vi "Queue Out Unitest.vi"(8 "error in":errorcluster, 11 "?":T1) -> (0 "error out":errorcluster, 3 "Quee Out":refnum<queue>)   [LabVIEW 2025]
uses:
  REF Enum Unitest.ctl
  support/Message Queue/LAB-IQ Message Queue.lvlib
  support/Message Queue/Message Cluster.ctl
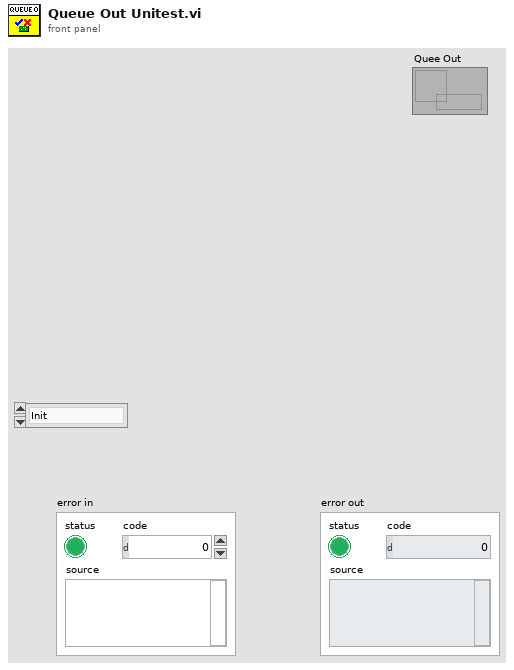
[diagram p1: front panel]
types:
  T1 = typedef "REF Enum Unitest.ctl" = enum16{"Init", "UI Loop", "LOAD COM LOOP", "HEAVE MOTOR COM LOOP", "SWAY MOTOR COM LOOP", "RAMP MOTOR COM LOOP", "TEMPERATURE COM LOOP", "HUMIDITY COM PORT", "ECR PORT", "MONITOR LOOP", "PROGRAM LOOP", "LOAD PID", "REPORT", "ACOUSTIC"}
  T2 = typedef "LAB-IQ Message Queue.lvlib/All Message Queues.ctl" = cluster{"UI Loop":refnum<queue>, "LOAD COM LOOP":refnum<queue>, "HEAVE MOTOR COM LOOP":refnum<queue>, "SWAY MOTOR COM LOOP":refnum<queue>, "RAMP MOTOR COM LOOP":refnum<queue>, "TEMPERATURE COM LOOP":refnum<queue>, "HUMIDITY COM PORT":refnum<queue>, "ECR PORT":refnum<queue>, "MONITOR LOOP":refnum<queue>, "PROGRAM LOOP":refnum<queue>, "LOAD PID":refnum<queue>, "REPORT":refnum<queue>, "ACOUSTIC":refnum<queue>}
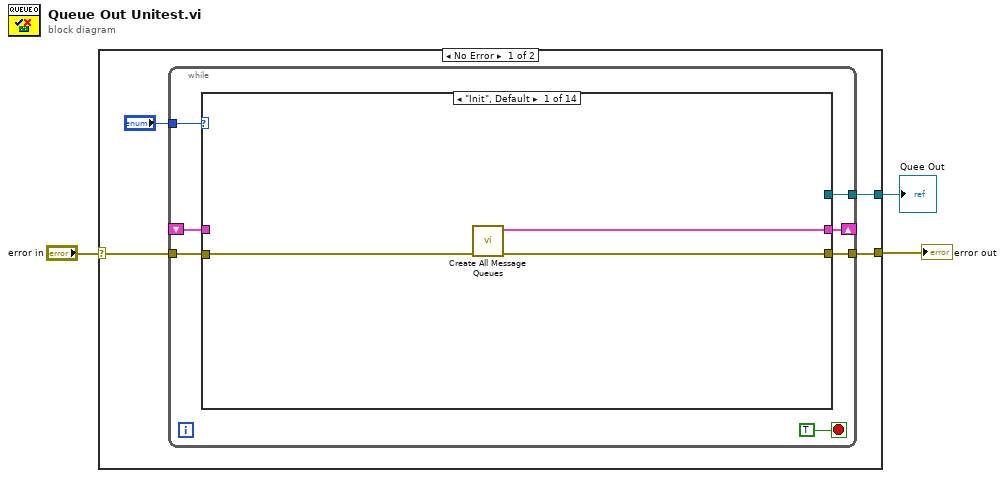
[diagram p0: block diagram]
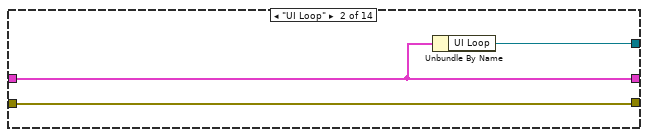
[diagram p2: hidden frame]
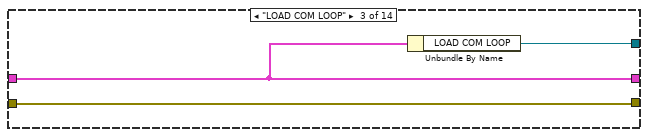
[diagram p3: hidden frame]
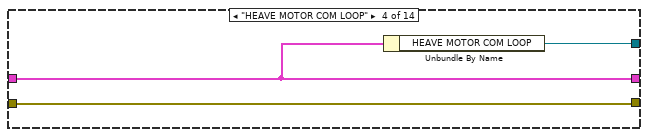
[diagram p4: hidden frame]
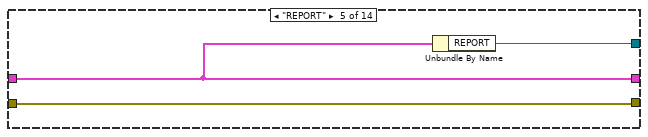
[diagram p5: hidden frame]
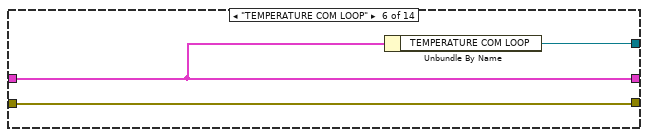
[diagram p6: hidden frame]
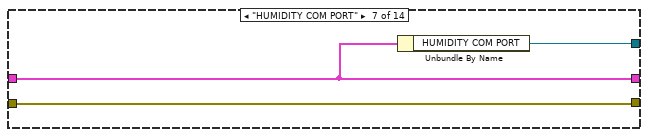
[diagram p7: hidden frame]
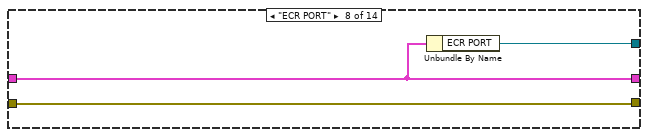
[diagram p8: hidden frame]
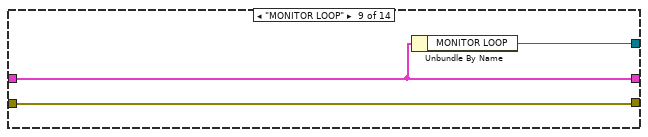
[diagram p9: hidden frame]
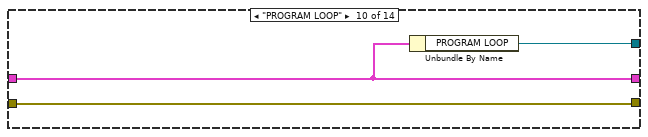
[diagram p10: hidden frame]
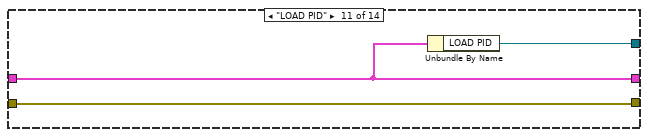
[diagram p11: hidden frame]
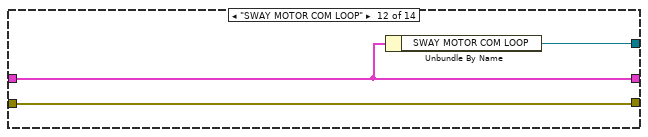
[diagram p12: hidden frame]
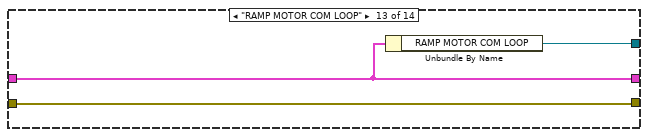
[diagram p13: hidden frame]
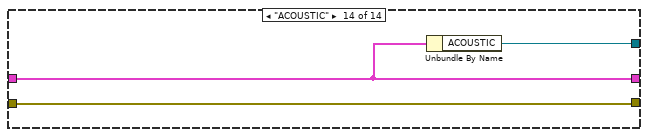
[diagram p14: hidden frame]
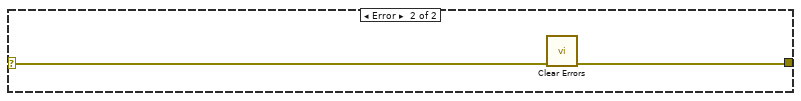
[diagram p15: hidden frame]
diagram:
  n1 = case shown="No Error" "error in" {
    selector: "error in" -> [w6 w58]
    tunnel: [w5 w57] -> w2
    tunnel: [w4 _] -> w1
    frame No Error {
      n2 = while {
        tunnel: "?" -> [w14]
        tunnel: w6 -> [w13]
        tunnel: [w12] -> w5
        shift-right: [w10] -> _
        shift-left: _ -> [w9]
        tunnel: [w8] -> w4
        stop <- TRUE stop-if-true
        n3 = case shown="\"Init\", Default" w14 {
          tunnel: w13 -> [w17 w20 w23 w26 w29 w32 w35 w38 w41 w44 w47 w50 w53 w56]
          tunnel: [w16 w20 w23 w26 w29 w32 w35 w38 w41 w44 w47 w50 w53 w56] -> w12
          tunnel: [w15 w19 w22 w25 w28 w30 w34 w37 w40 w43 w46 w49 w52 w55] -> w10
          tunnel: w9 -> [_ w19 w22 w25 w28 w30 w34 w37 w40 w43 w46 w49 w52 w55]
          tunnel: [_ w18 w21 w24 w27 w31 w33 w36 w39 w42 w45 w48 w51 w54] -> w8
          frame "Init", Default {
            n4 = call "Create All Message Queues.vi"("error in (no error)"=w17) -> ("error out"=w16:errorcluster, "Message Queues out"=w15:T2)  [unwired: 9 in]
          }
          frame "UI Loop" {
            n5 = Unbundle By Name(w19) -> ("UI Loop"=w18:refnum<queue>)
          }
          frame "LOAD COM LOOP" {
            n6 = Unbundle By Name(w22) -> ("LOAD COM LOOP"=w21:refnum<queue>)
          }
          frame "HEAVE MOTOR COM LOOP" {
            n7 = Unbundle By Name(w25) -> ("HEAVE MOTOR COM LOOP"=w24:refnum<queue>)
          }
          frame "REPORT" {
            n8 = Unbundle By Name(w28) -> ("REPORT"=w27:refnum<queue>)
          }
          frame "TEMPERATURE COM LOOP" {
            n9 = Unbundle By Name(w30) -> ("TEMPERATURE COM LOOP"=w31:refnum<queue>)
          }
          frame "HUMIDITY COM PORT" {
            n10 = Unbundle By Name(w34) -> ("HUMIDITY COM PORT"=w33:refnum<queue>)
          }
          frame "ECR PORT" {
            n11 = Unbundle By Name(w37) -> ("ECR PORT"=w36:refnum<queue>)
          }
          frame "MONITOR LOOP" {
            n12 = Unbundle By Name(w40) -> ("MONITOR LOOP"=w39:refnum<queue>)
          }
          frame "PROGRAM LOOP" {
            n13 = Unbundle By Name(w43) -> ("PROGRAM LOOP"=w42:refnum<queue>)
          }
          frame "LOAD PID" {
            n14 = Unbundle By Name(w46) -> ("LOAD PID"=w45:refnum<queue>)
          }
          frame "SWAY MOTOR COM LOOP" {
            n15 = Unbundle By Name(w49) -> ("SWAY MOTOR COM LOOP"=w48:refnum<queue>)
          }
          frame "RAMP MOTOR COM LOOP" {
            n16 = Unbundle By Name(w52) -> ("RAMP MOTOR COM LOOP"=w51:refnum<queue>)
          }
          frame "ACOUSTIC" {
            n17 = Unbundle By Name(w55) -> ("ACOUSTIC"=w54:refnum<queue>)
          }
        }
      }
    }
    frame Error {
      n18 = call <vilib>:"Clear Errors.vi"("error in (no error)"=w58) -> ("error out"=w57:errorcluster)  [unwired: 5 in, 1 out]
    }
  }
  "error out" <- w2
  "Quee Out" <- w1
